vi "Edit a Button--Material.vi"() -> ()   [LabVIEW 2021]
doc: "Edit/create buttons based on a few built-in templates.\n\n<b>Code Developed By:</b>\nTechnology Service Corporation\n1983 S Liberty Drive\nBloomington, IN 47403\nPhone: 812 558-7100\nwww.tsc.com/atcs\n\nDeveloper:\nDaniel Coons"
uses:
  <vilib>/Utility/miscctls.llb/LVPositionTypeDef.ctl
  user32.dll
  Material Theme/Material Theme.lvclass
  Material-Scheme/Material-Scheme.lvclass
panel:
  in  "Color Level":u16(ring) items=["Primary", "Secondary", "Tertiary", "Error", "Primary Fixed", "Secondary Fixed", "Tertiary Fixed"]
  in  "Theme":u16(ring) items=["Light Theme", "Light Medium Contrast", "Light High Contrast", "Dark Theme", "Dark Medium Contrast", "Dark High Constrast"]
  in  "theme path":path
  in  "Open":bool
  in  "Button Type":u16(ring) items=["FAB--icon--rounded.ctl", "filled--icon--rectangular.ctl", "filled--icon--rounded.ctl", "filled--text--rectangular.ctl", "filled--text--rounded.ctl", "nooutline--icon--rectangular--40x40.ctl", "nooutline--icon--rectangular.ctl", "nooutline--icon--rounded.ctl", "nooutline--text--rectangular.ctl", "nooutline--text--rounded.ctl", "outline--icon--rectangular.ctl", "outline--icon--rounded.ctl", "outline--text--rectangular.ctl", "outline--text--rounded.ctl", "tonal--icon--rectangular.ctl", "tonal--icon--rounded.ctl", "tonal--text--rectangular.ctl", "tonal--text--rounded.ctl"]
  in  "Tab Control":enum32{"Button Formatting"}(tab)
  in  "Image Color":u32(colorbox)=3563918
  in  "update button text location":bool
  in  "Button Text Location":cluster{"Left":i32, "Top":i32}
  in  "update button size":bool
  in  "Button Size":cluster{"Width":u32, "Height":u32}={"Width"=204, "Height"=48}
  in  "update colors":bool
  in  "Boolean Text":string
  in  "Boolean Text Format":T1={"Font:Color"=3563918, "Font:Bold?"=TRUE, "Font:Name"="App Font", "Font:Size"=22}
  in  "Boolean Colors":T2={"false color"={"border"=15922170, "fill"=15922170}, "true color"={"border"=14936305, "fill"=14936305}, "click false color"={"border"=14410221, "fill"=14410221}, "click true color"={"border"=14410221, "fill"=14410221}, "hover false color"={"border"=14540516, "fill"=14540516}, "hover true color"={"border"=14540516, "fill"=14540516}}
  in  "update text format":bool
  in  "Decal Image":path
  out "b":u8
  out "g":u8
  out "r":u8
  out "Color":u32(colorbox)
  in  "Hex Color":u32 max=16777215 format="%06x"
  in  "close":bool
  out "header":bool
  in  "Save":bool
  out "error out":errorcluster
  # "if using hex colors, put in the value and copy/paste\nto whichever desired color box"
  # "Note: match the size of the replacement\nimage so scaling is correct (default 24x24)\n\nFor other desired sizes, save the control and\nopen it in LabVIEW. Click the Wrench in the\ntool bar to change to Edit Mode. \n\nRight click the image on the button and \nchoose Original Size.\n\nGetting the right size glyph can be a\nchallenge with customized buttons"
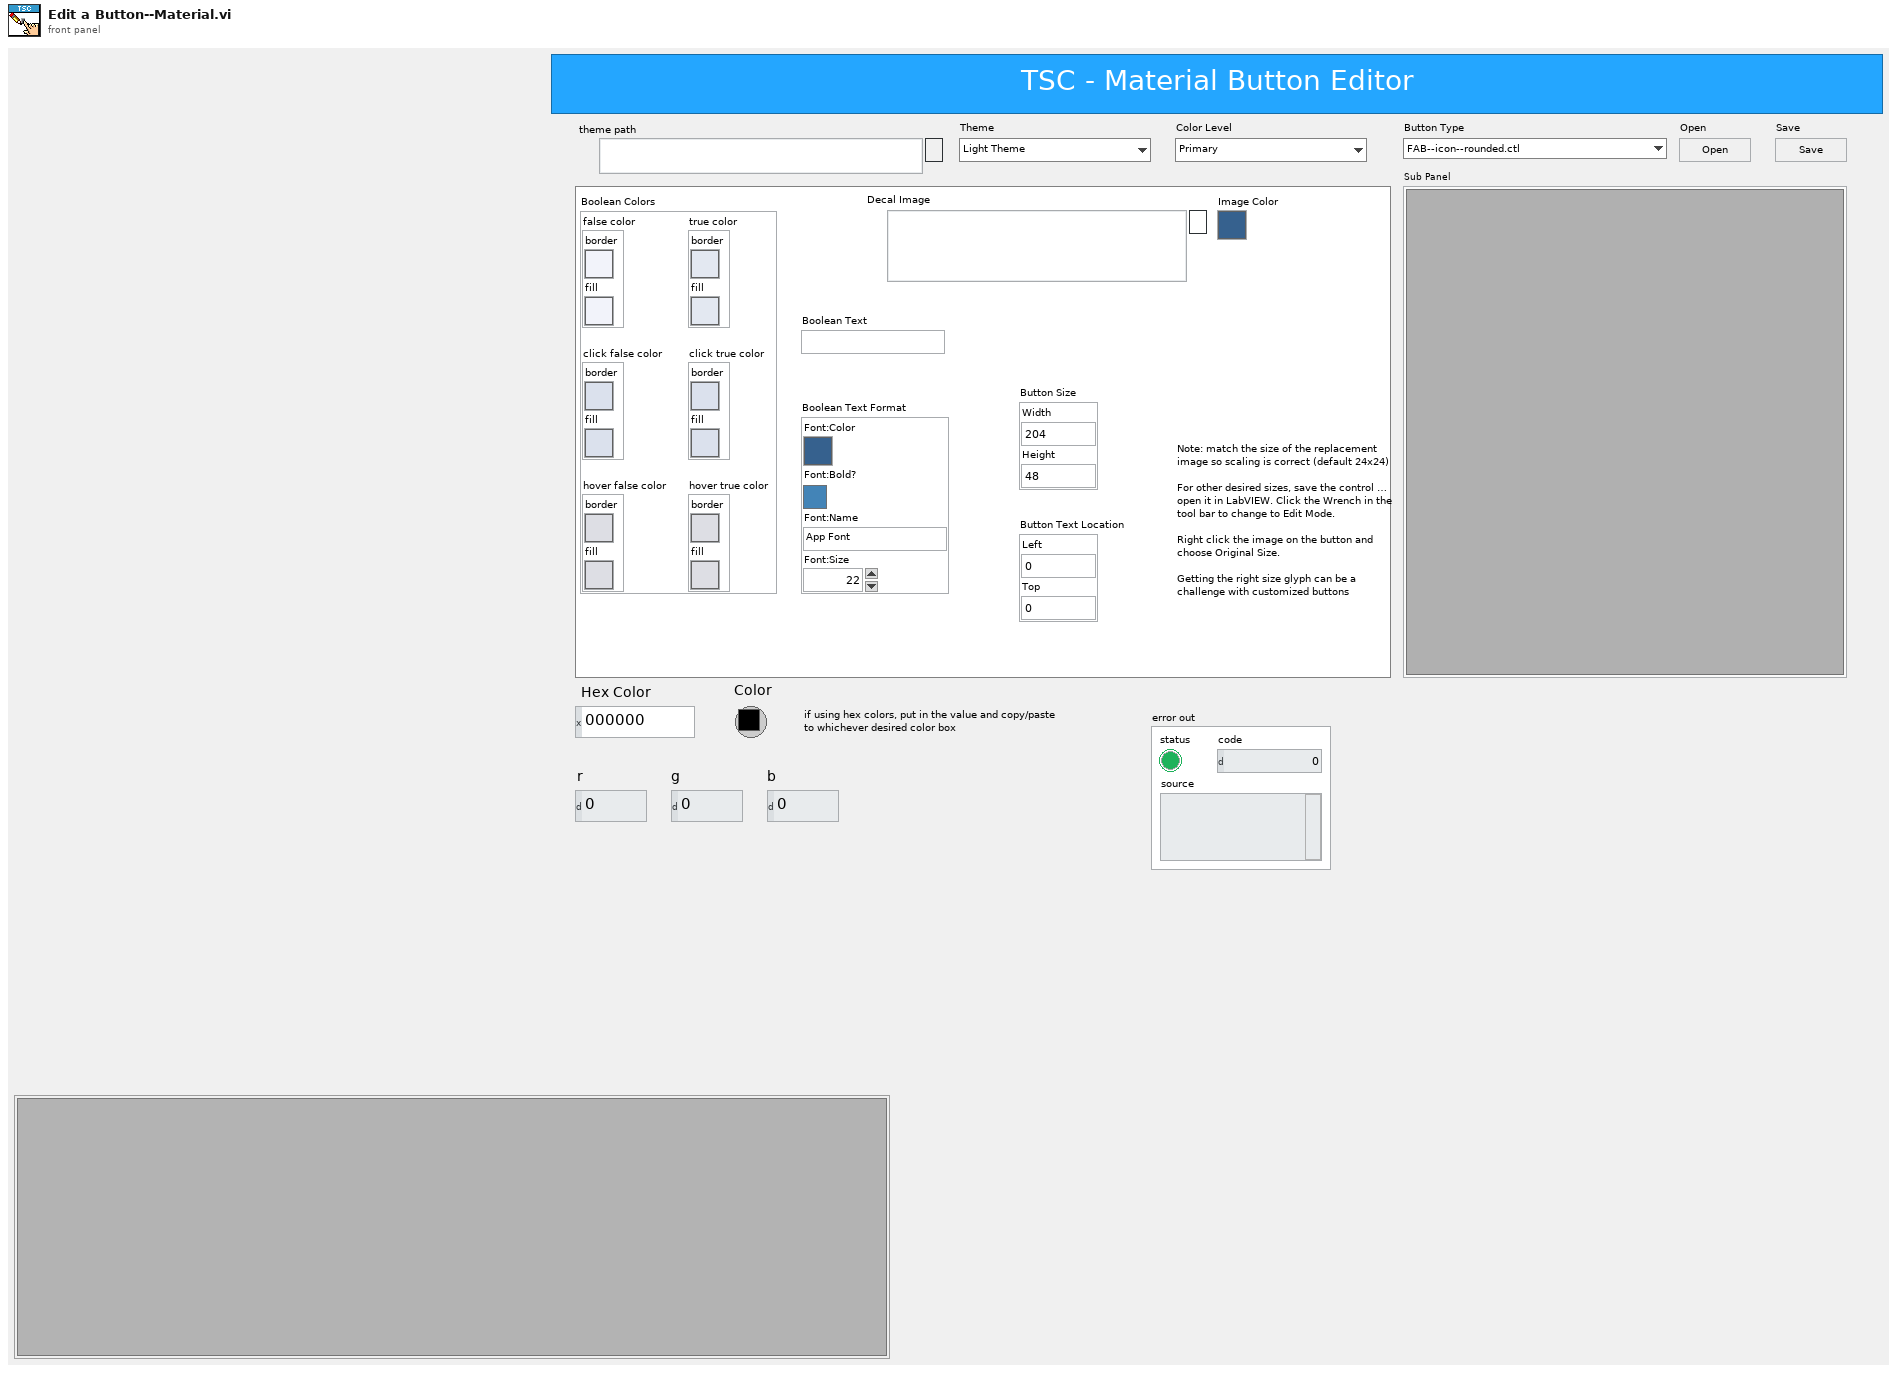
[diagram p1: front panel]
types:
  T1 = cluster{"Font:Color":u32, "Font:Bold?":bool, "Font:Name":string, "Font:Size":u32}
  T2 = cluster{"false color":cluster{"border":u32, "fill":u32}, "true color":cluster{"border":u32, "fill":u32}, "click false color":cluster{"border":u32, "fill":u32}, "click true color":cluster{"border":u32, "fill":u32}, "hover false color":cluster{"border":u32, "fill":u32}, "hover true color":cluster{"border":u32, "fill":u32}}
  T3 = typedef "User Events.ctl" = cluster{"update colors":refnum<user-event>, "update boolean data":refnum<user-event>, "update image":refnum<user-event>}
  T4 = typedef "LVPositionTypeDef.ctl" = cluster{"Left":i32, "Top":i32}
  T5 = enum32{"invalid VI type", "Standard VI", "Control VI", "Global VI", "Polymorphic VI", "Configuration VI", "SubSystem", "Facade VI", "Method VI", "Statechart Diagram VI"}
  T6 = typedef "LVBoundsTypeDef.ctl" = cluster{"Width":u32, "Height":u32}
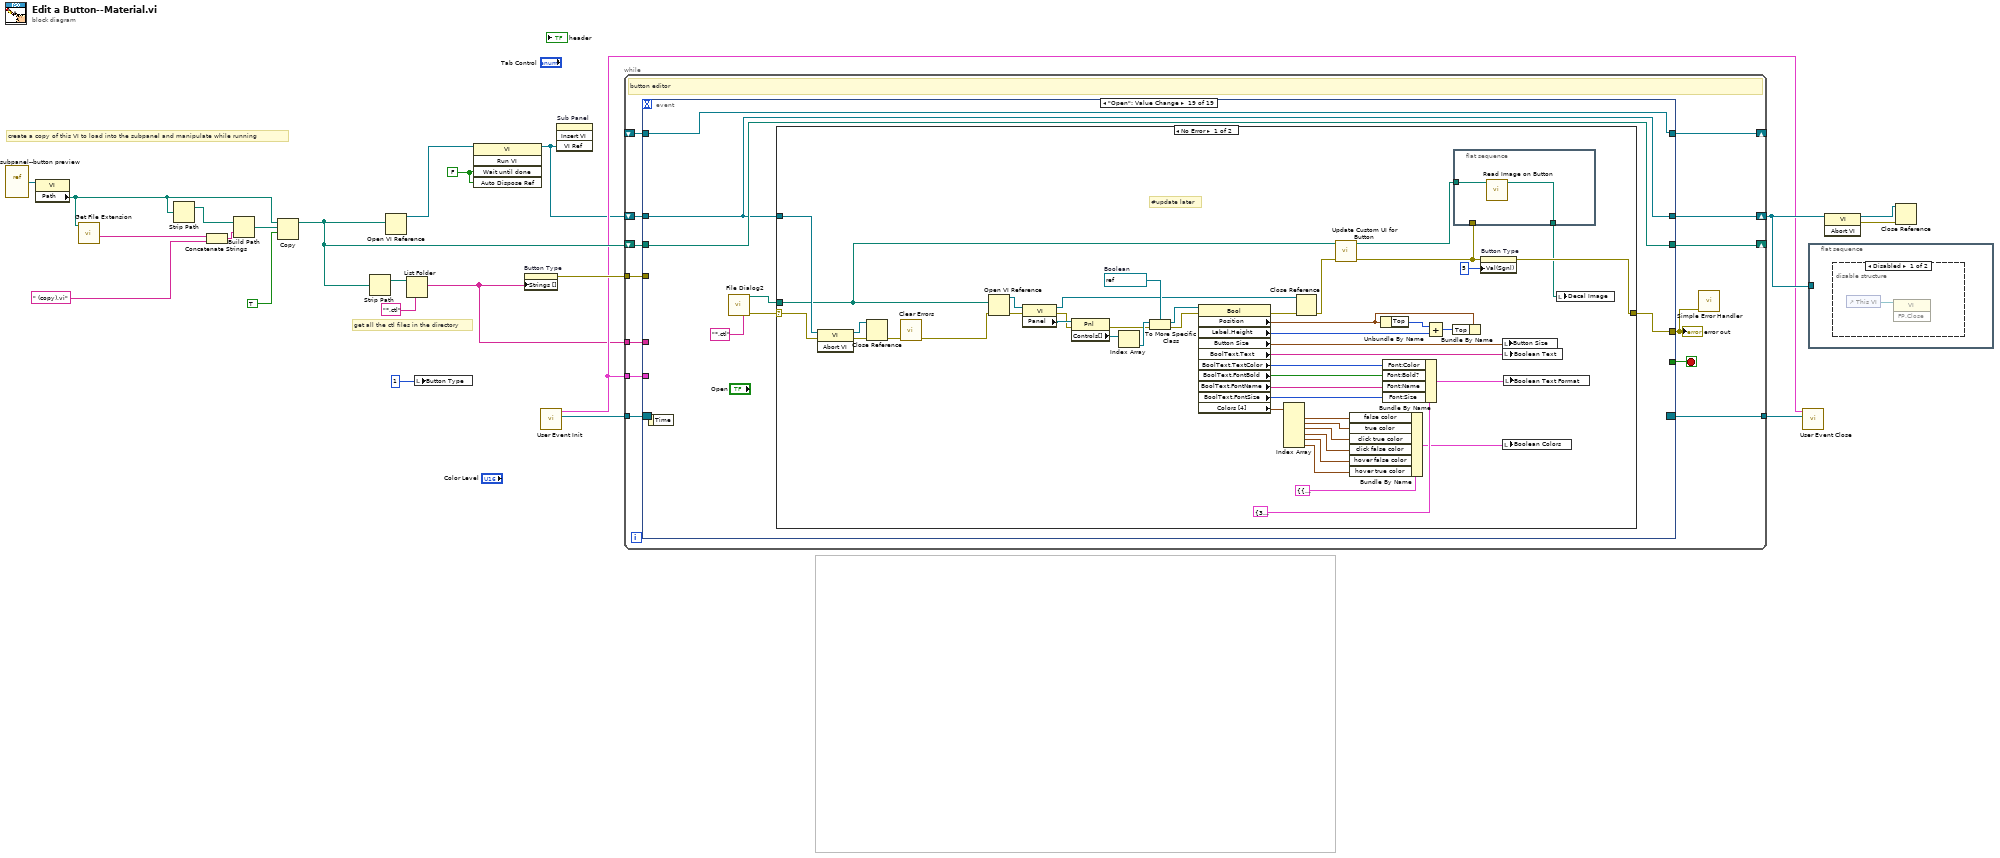
[diagram p0: block diagram]
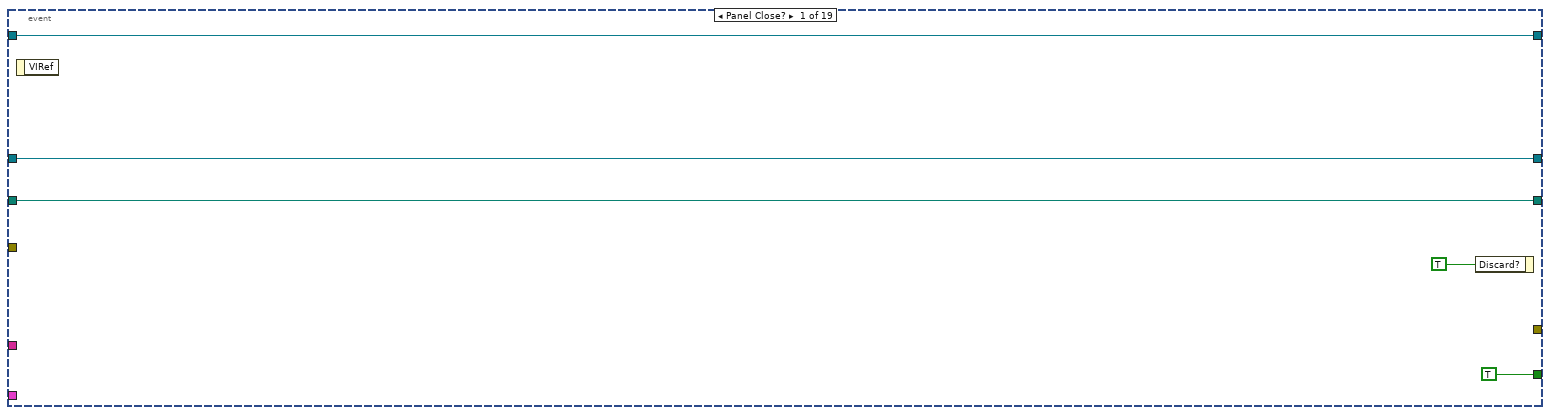
[diagram p3: hidden frame]
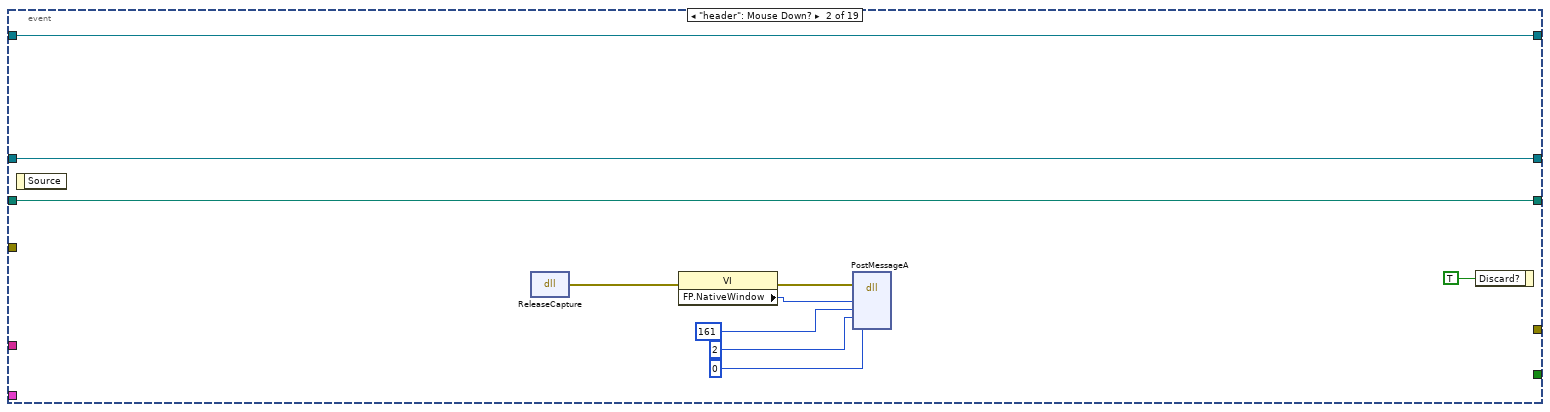
[diagram p4: hidden frame]
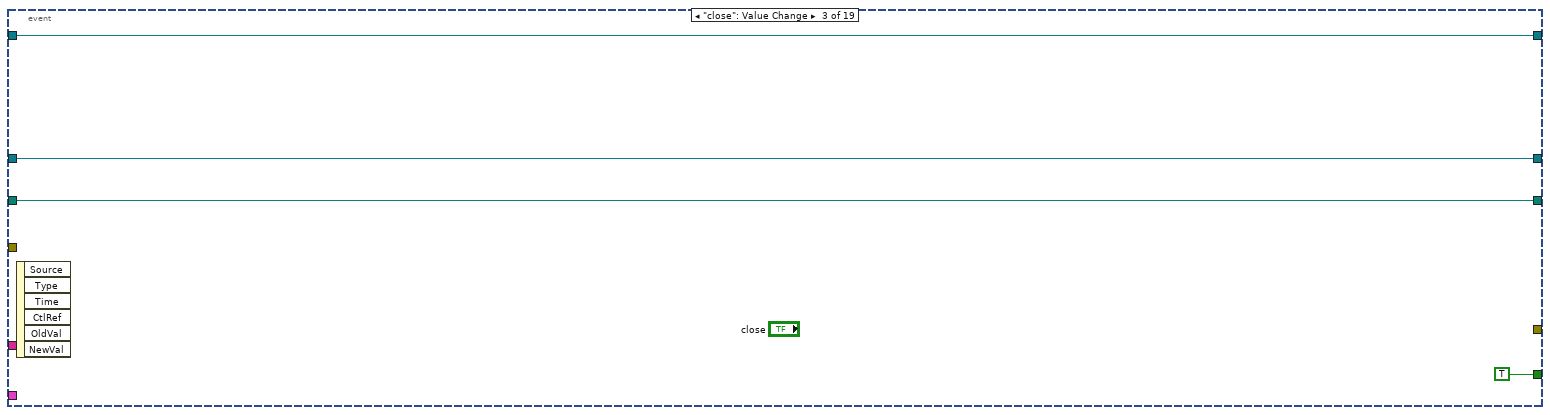
[diagram p5: hidden frame]
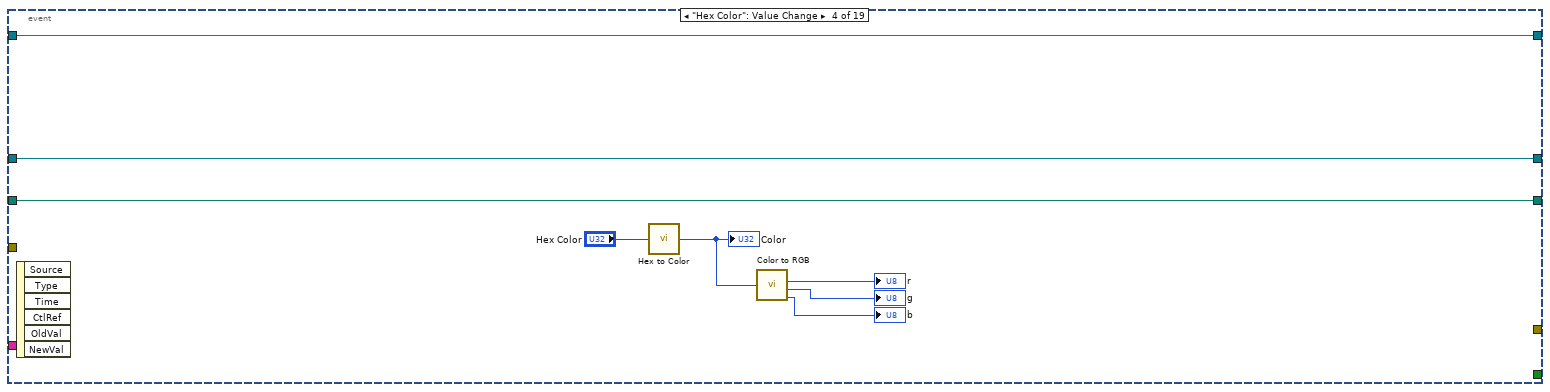
[diagram p6: hidden frame]
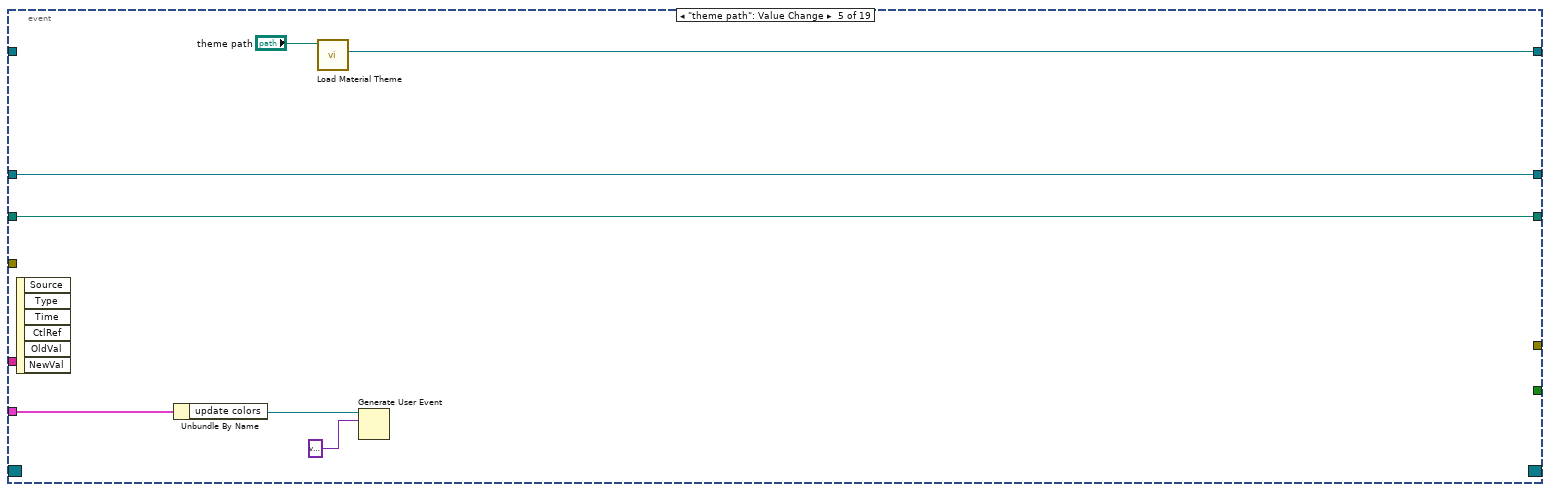
[diagram p7: hidden frame]
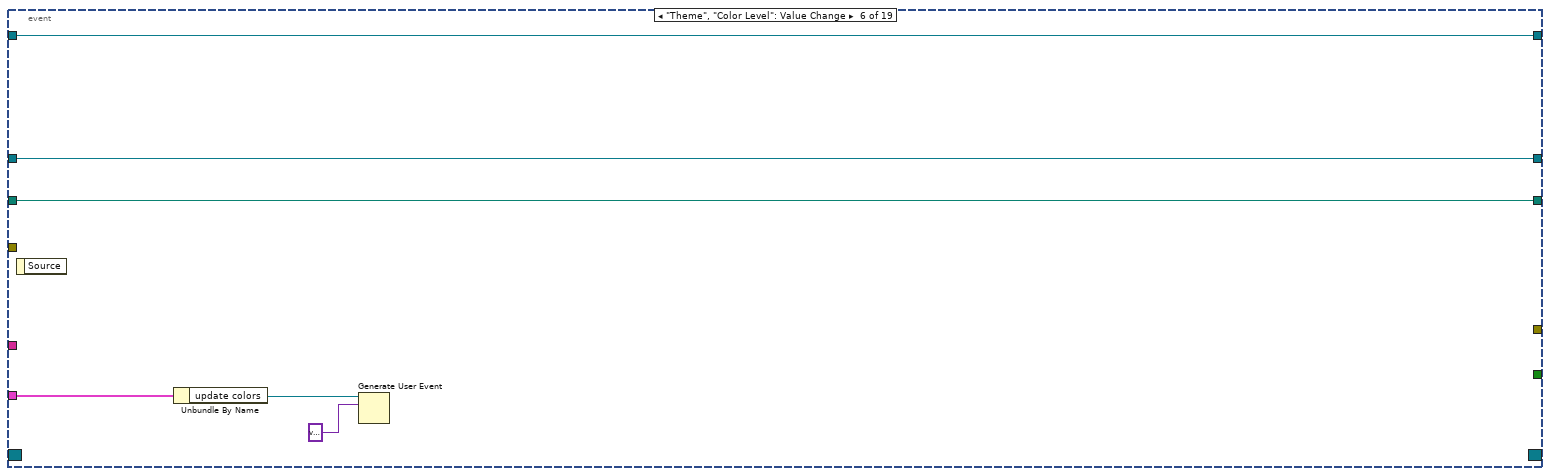
[diagram p8: hidden frame]
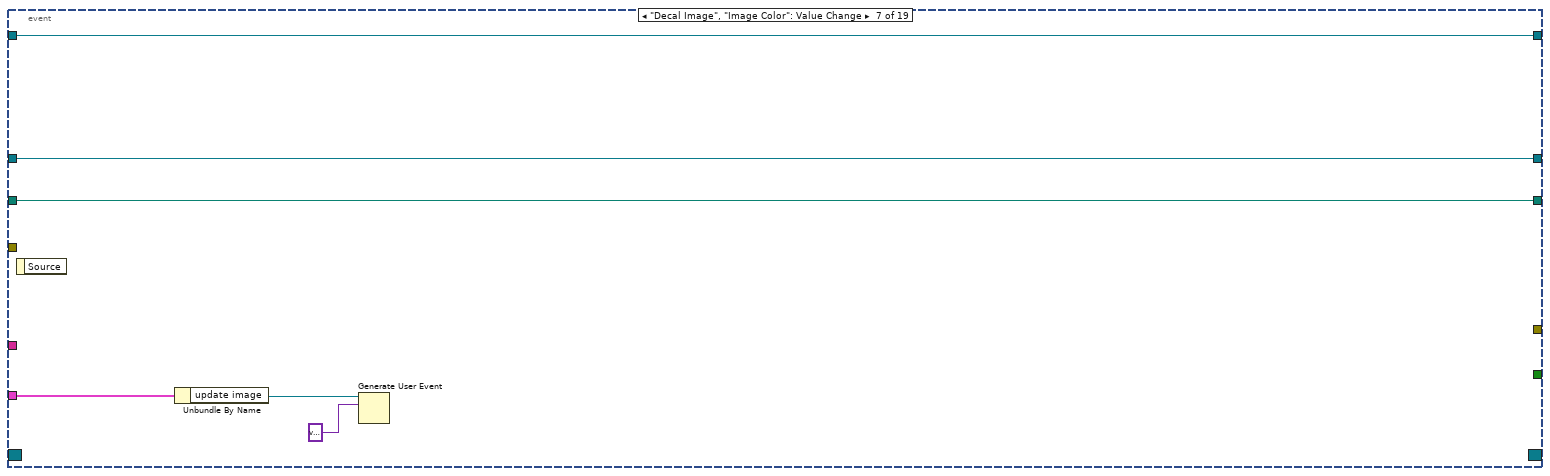
[diagram p9: hidden frame]
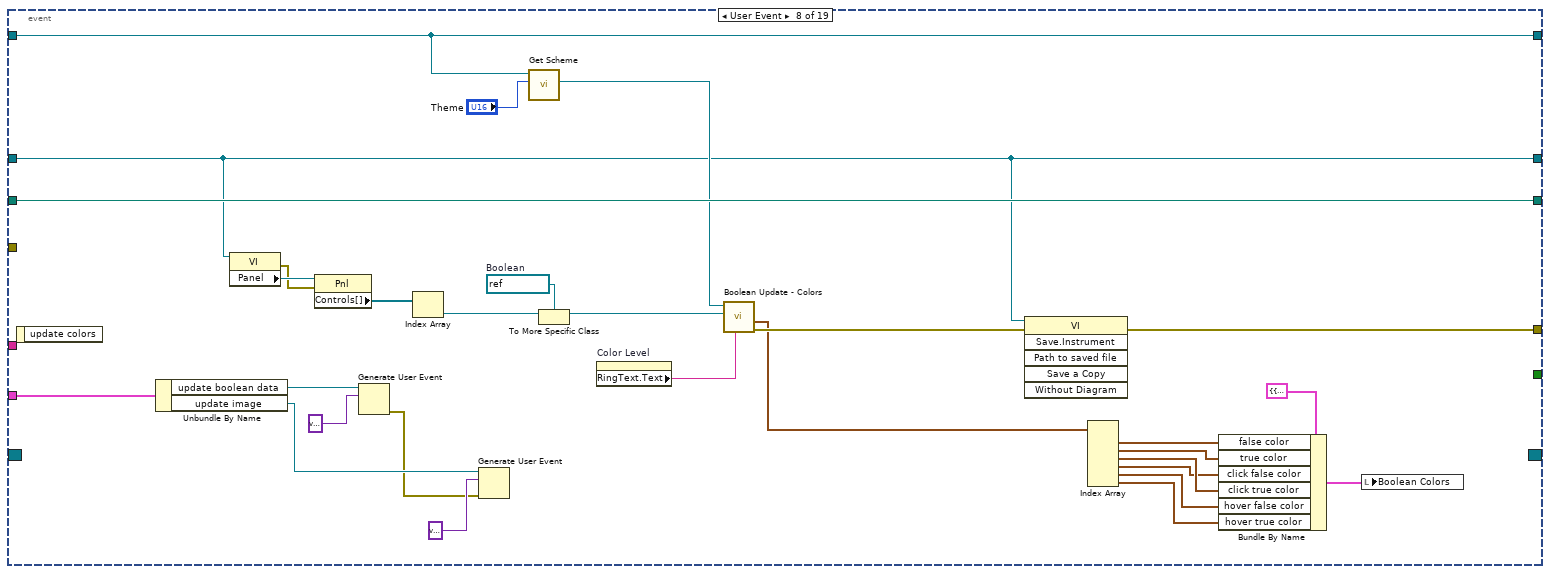
[diagram p10: hidden frame]
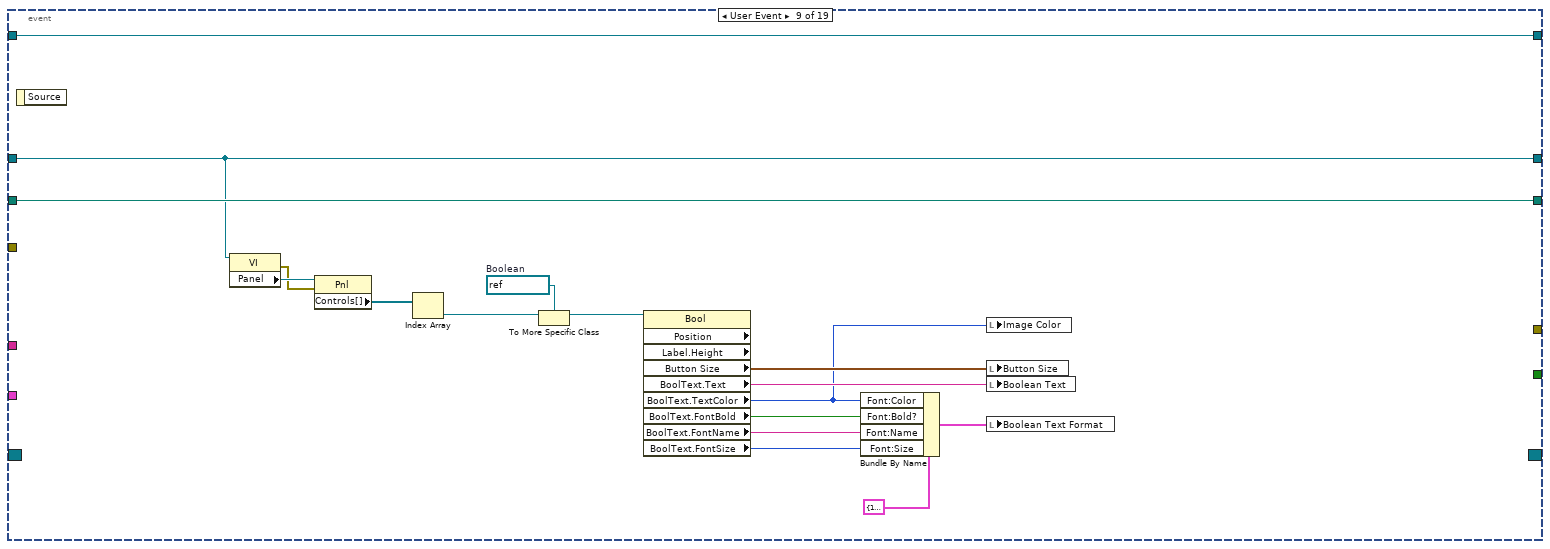
[diagram p11: hidden frame]
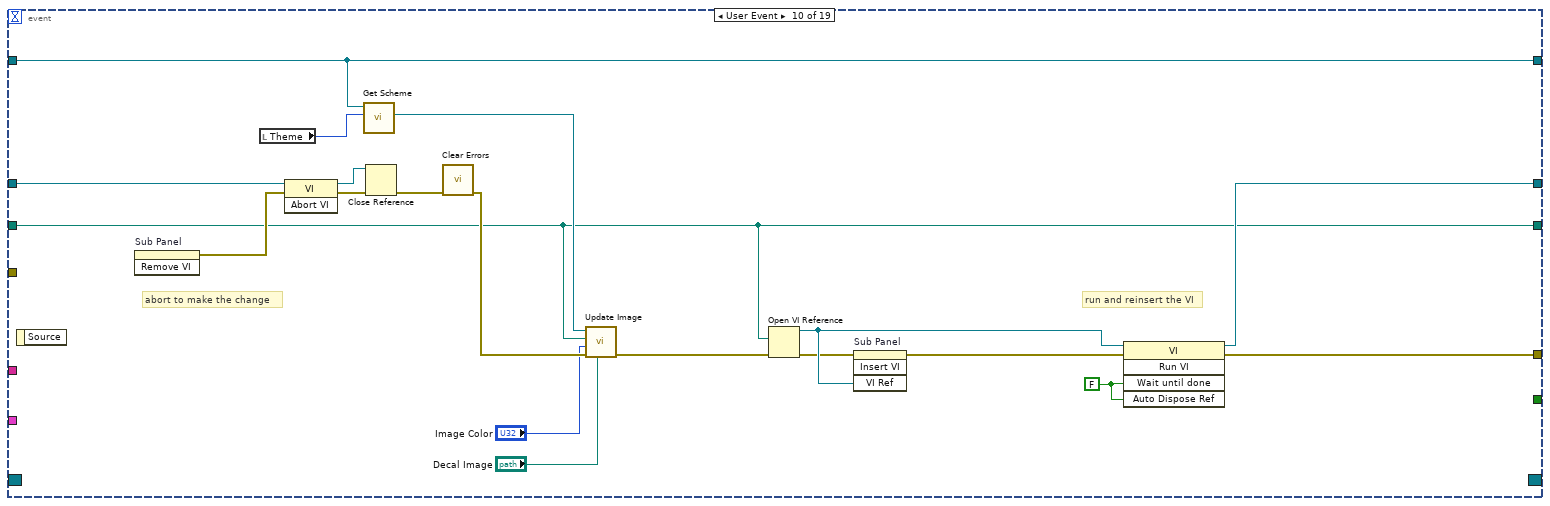
[diagram p12: hidden frame]
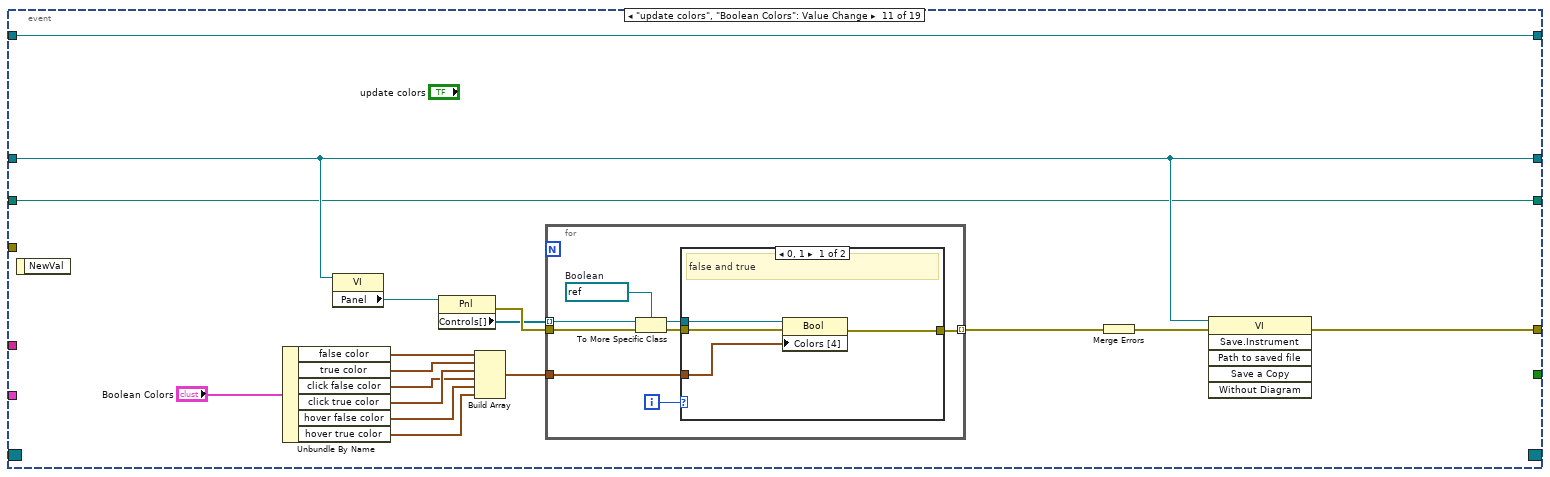
[diagram p13: hidden frame]
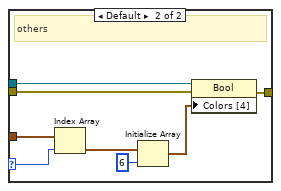
[diagram p14: hidden frame]
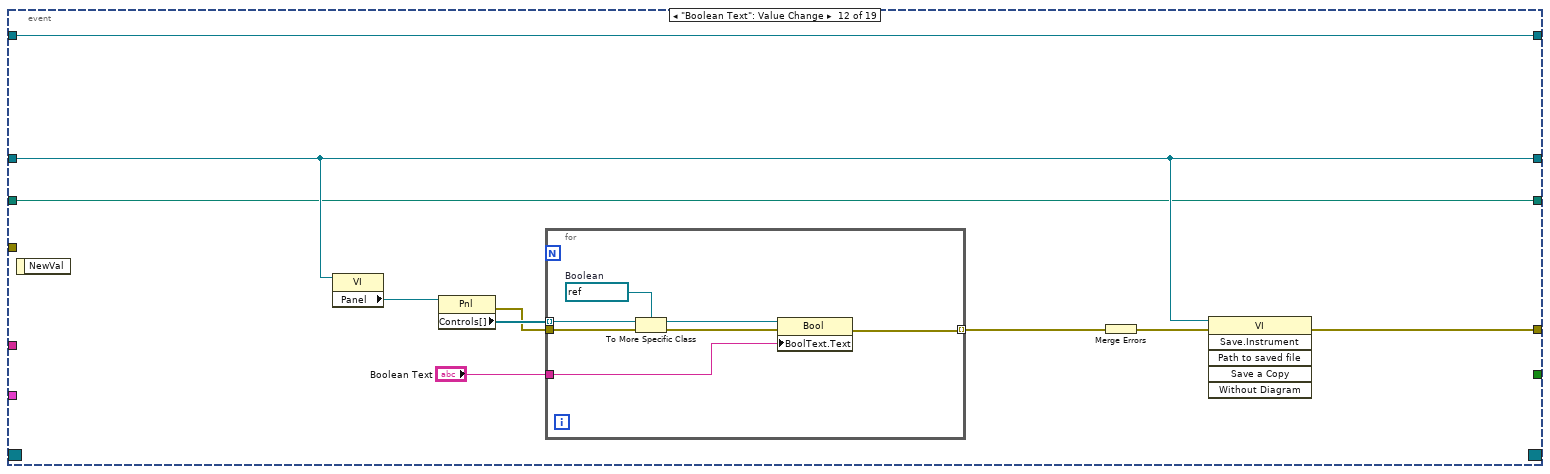
[diagram p15: hidden frame]
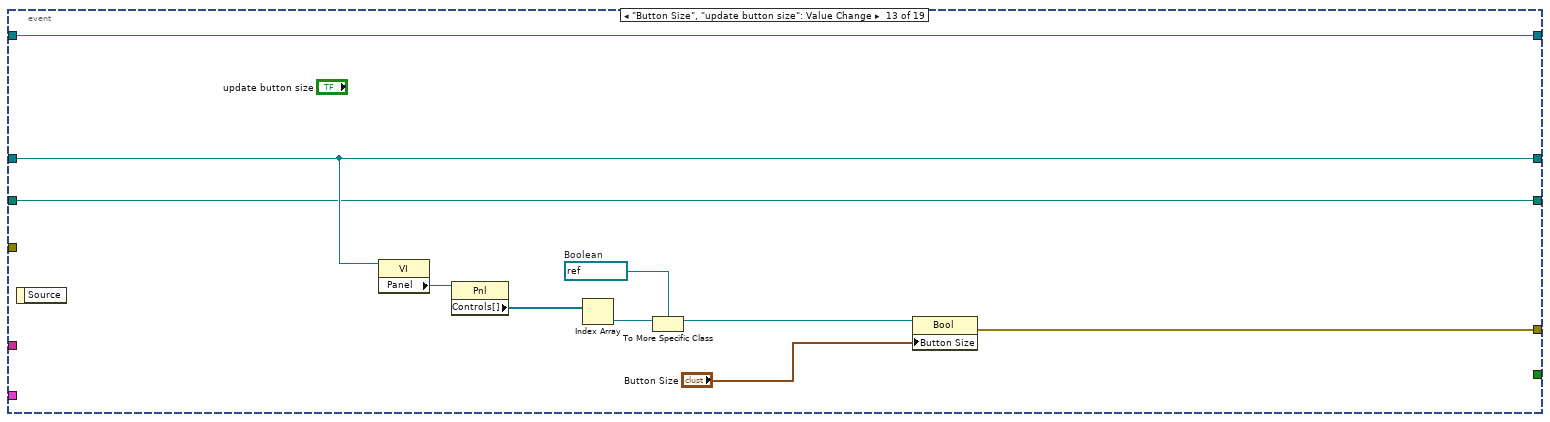
[diagram p16: hidden frame]
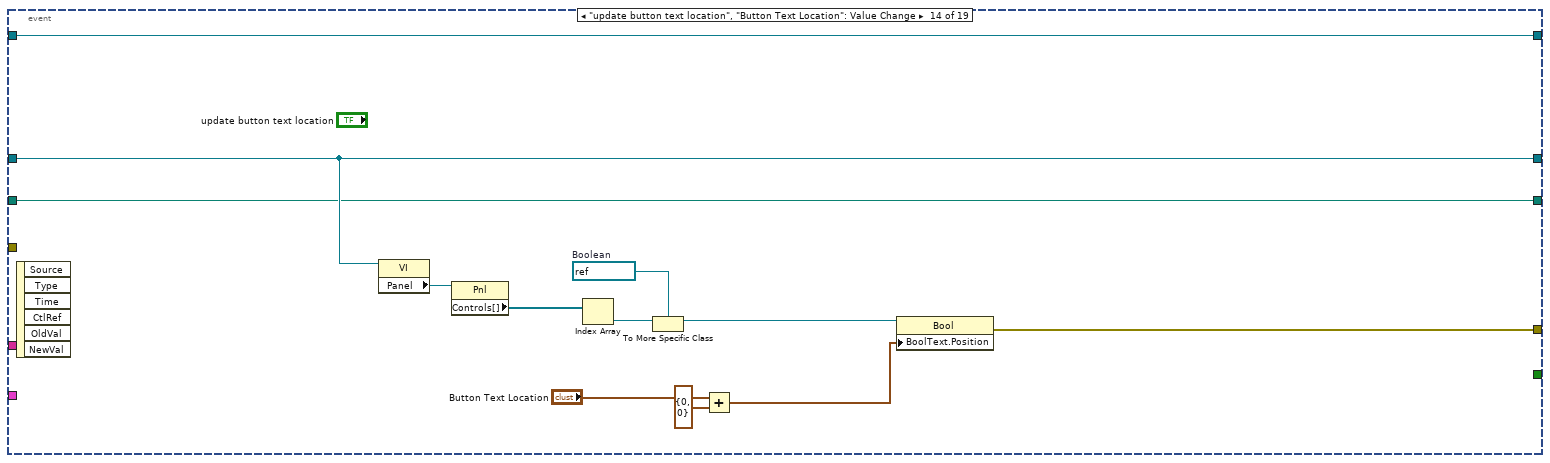
[diagram p17: hidden frame]
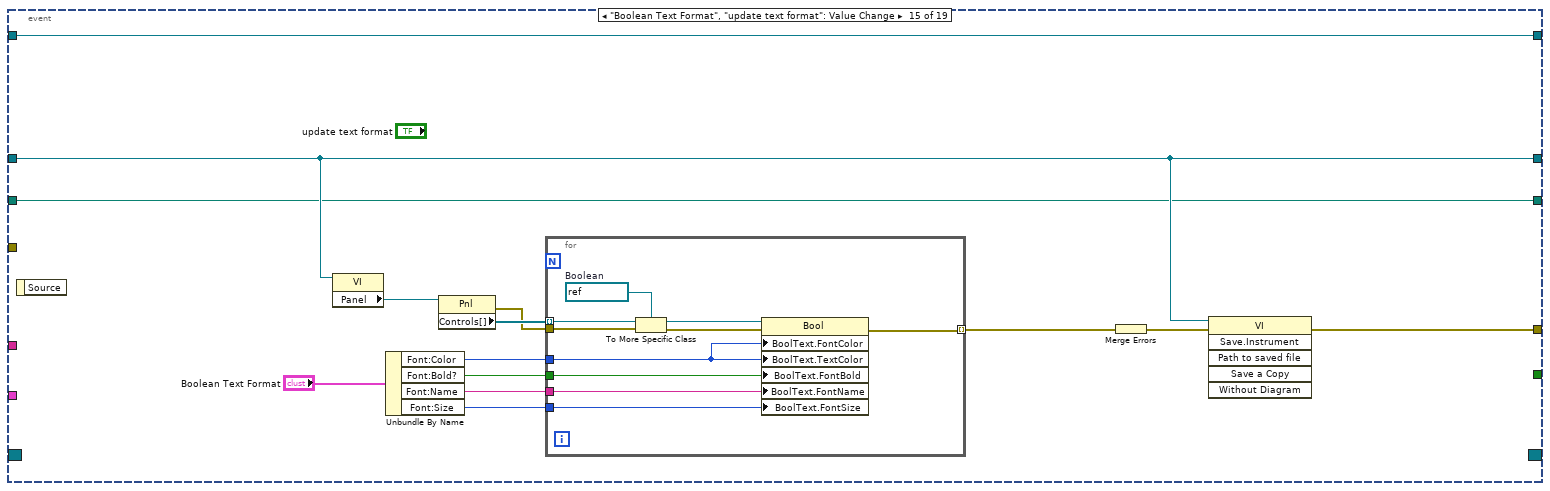
[diagram p18: hidden frame]
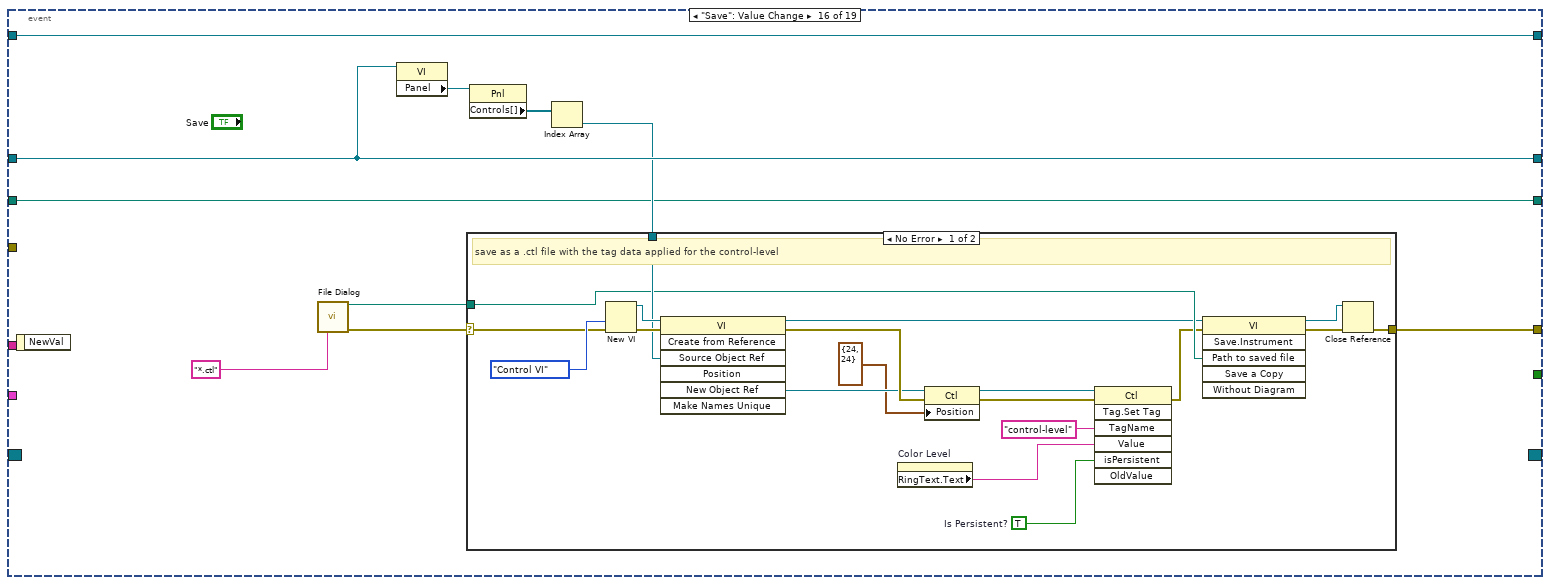
[diagram p19: hidden frame]
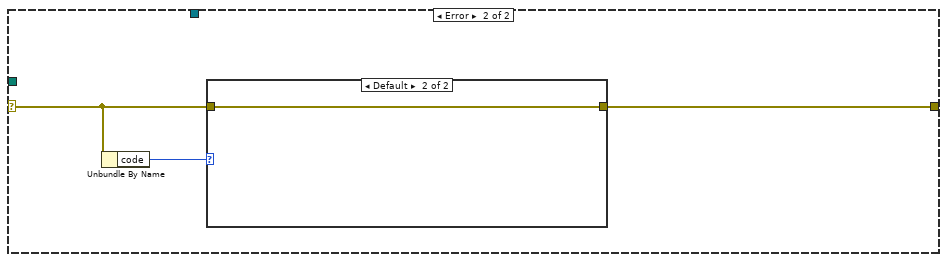
[diagram p20: hidden frame]
diagram:
  w12 = FALSE ("Activate?")
  # "get all the ctl files in the directory"
  # "create a copy of this VI to load into the subpanel and manipulate while running"
  n1 = vi-ref "subpanel--button preview.vi"() -> (w10:refnum<vi>)
  n2 = property class="VI"(reference=w10) -> ("Path"=w3:path)  [unwired: 1 in, 2 out]
  n3 = call <vilib>:"Get File Extension.vi"("file"=w3) -> ("filename without extension"=w4:string)  [unwired: 6 in, 4 out]
  n4 = Strip Path(path=w3) -> (stripped path=w6:path)  [unwired: 1 out]
  n5 = Concatenate Strings(w4, " (copy).vi" ("string")) -> (w7:string)
  n6 = Build Path(base path=w6, name or relative path=w7) -> (appended path=w5:path)
  n7 = Copy(9:TRUE ("overwrite (F)"), 10:w5, 11:w3) -> (3:w17:path)  [unwired: 2 in, 2 out]
  n8 = Strip Path(path=w17) -> (stripped path=w18:path)  [unwired: 1 out]
  n9 = Open VI Reference(vi path=w17) -> (vi reference=w16:refnum<vi>)  [unwired: 5 in, 1 out]
  n10 = List Folder(path=w18, pattern="*.ctl") -> (filenames=w11:string[])  [unwired: 2 in, 3 out]
  n11 = local write "Button Type"(1) -> ()
  n12 = invoke class="VI" method="Run VI"(reference=w16, "Wait until done"=w12, "Auto Dispose Ref"=w12) -> (reference out=w1:refnum<vi>)  [unwired: 2 in, 4 out]
  n13 = property on="Button Type" class="Ring (strict)"("Strings []"=w11) -> (error out=w21:errorcluster)  [unwired: 2 in, 1 out]
  n14 = call "User Event Init.vi"() -> ("Event Registration Refnum"=w15:refnum<event-registration>, "user events"=w13:T3)  [unwired: 10 in]
  n15 = invoke on="Sub Panel" class="SubPnl" method="Insert VI"("VI Ref"=w1) -> ()  [unwired: 3 in, 4 out]
  n16 = while {
    shift-right: [w34] -> w20
    shift-left: w1 -> [w35]
    shift-right: [w32] -> _
    shift-left: w17 -> [w33]
    tunnel: w21 -> [w31]
    shift-right: [w30] -> _
    shift-left: _ -> [w29]
    tunnel: w15 -> [w28]
    tunnel: [w27] -> w14
    tunnel: w13 -> [w26]
    tunnel: w11 -> [w25]
    stop <- w36 stop-if-true
    # "button editor"
    n17 = event shown="[18] \"Open\": Value Change" {
      selector: w28 -> [_ _ _ _ _ _ _ _ _ _ _ _ _ _ _ _ _ _ _]
      dyn-events: [_ _ _ _ _ _ _ _ _ _ _ _ _ _ _ _ _ _ _] -> w27
      timeout: _ -> [_ _ _ _ _ _ _ _ _ _ _ _ _ _ _ _ _ _ _]
      tunnel: [TRUE _ TRUE _ _ _ _ _ _ _ _ _ _ _ _ _ _ _ _] -> w36
      tunnel: w35 -> [w39 w51 w54 w63 w67 w75 w81 w88 w121 w147 w160 w187 w207 w219 w231 w256 w285 w339 w350]
      tunnel: [w39 w51 w54 w63 w67 w75 w81 w88 w121 w140 w160 w187 w207 w219 w231 w256 w285 w332 w350] -> w34
      tunnel: [_ _ _ _ _ _ _ w86 _ w129 w159 w188 w205 w217 w232 w253 w284 w333 w352] -> w24
      tunnel: w33 -> [w38 w43 w53 w57 w70 w76 w82 w111 w128 w131 w149 w186 w203 w214 w225 w249 w283 w331 w355]
      tunnel: [w38 w43 w53 w57 w70 w76 w82 w111 w128 w131 w149 w186 w203 w214 w225 w249 w283 w331 w355] -> w32
      tunnel: w31 -> [_ _ _ _ _ _ _ _ _ _ _ _ _ _ _ _ _ _ _]
      tunnel: [w37 w42 w52 w56 w68 w72 w78 w102 w127 w144 w148 w185 w202 w213 w224 w248 w282 w337 w349] -> w30
      tunnel: w29 -> [w37 w42 w52 w56 _ w72 w78 w102 w127 w144 w148 w185 w202 w213 w224 w248 w282 w337 w349]
      tunnel: w26 -> [_ _ _ _ w66 w74 w80 w89 _ _ _ _ _ _ _ _ _ w319 _]
      tunnel: w25 -> [_ _ _ _ _ _ _ _ _ _ _ _ _ _ _ _ _ _ _]
      event Panel Close? {
        n18 = event-data() -> ()  [unwired: 1 in, 1 out]
        n19 = event-data("Discard?"=TRUE) -> ()  [unwired: 1 in, 1 out]
      }
      event "header": Mouse Down? {
        n20 = event-data() -> ()  [unwired: 1 in, 1 out]
        n21 = dll-call lib="user32.dll" fn="ReleaseCapture"() -> (error out=w46:errorcluster)  [unwired: 4 in, 1 out]
        n22 = property class="VI"(error in=w46) -> (error out=w45:errorcluster, "FP.NativeWindow"=w44:u64)  [unwired: 1 in, 1 out]
        n23 = dll-call lib="user32.dll" fn="PostMessageA"(error in=w45, "hWnd"=w44, "Msg"=161, "wParam"=2, "lParam"=0) -> ()  [unwired: 7 in, 2 out]
        n24 = event-data("Discard?"=TRUE) -> ()  [unwired: 1 in, 1 out]
      }
      event "close": Value Change {
        n25 = event-data() -> ()  [unwired: 1 in, 6 out]
      }
      event "Hex Color": Value Change {
        n26 = event-data() -> ()  [unwired: 1 in, 6 out]
        n27 = call <vilib>:"Hex to Color.vi"("Hex String"="Hex Color") -> ("Color Box"=w61:u32)  [unwired: 4 in]
        "Color" <- w61
        n28 = call <vilib>:"Color to RGB.vi"("Color"=w61) -> ("R"=→"r":u8, "G"=→"g":u8, "B"=→"b":u8)  [unwired: 1 out]
      }
      event "theme path": Value Change {
        n29 = event-data() -> ()  [unwired: 1 in, 6 out]
        n30 = Unbundle By Name(w66) -> ("update colors"=w64:refnum<user-event>)
        n31 = call "Load Material Theme.vi"("file path (use dialog)"="theme path") -> ("Theme"=w68:refnum<class "Material Theme.lvclass">)  [unwired: 9 in, 1 out]
        n32 = Generate User Event(user event=w64, event data cluster=variant ("event data")) -> ()  [unwired: 2 in, 2 out]
      }
      event "Theme", "Color Level": Value Change {
        n33 = event-data() -> ()  [unwired: 1 in, 1 out]
        n34 = Unbundle By Name(w74) -> ("update colors"=w71:refnum<user-event>)
        n35 = Generate User Event(user event=w71, event data cluster=variant ("event data")) -> ()  [unwired: 2 in, 2 out]
      }
      event "Decal Image", "Image Color": Value Change {
        n36 = event-data() -> ()  [unwired: 1 in, 1 out]
        n37 = Unbundle By Name(w80) -> ("update image"=w77:refnum<user-event>)
        n38 = Generate User Event(user event=w77, event data cluster=variant ("event data")) -> ()  [unwired: 2 in, 2 out]
      }
      event User Event {
        w105 = refnum<vi> refnum  # Boolean
        n39 = event-data() -> ()  [unwired: 1 in, 1 out]
        n40 = Unbundle By Name(w89) -> ("update boolean data"=w91:refnum<user-event>, "update image"=w84:refnum<user-event>)
        n41 = property class="VI"(reference=w88) -> (error out=w107:errorcluster, "Panel"=w110:refnum<vi>)  [unwired: 1 in, 1 out]
        n42 = property class="Pnl"(reference=w110, error in=w107) -> ("Controls[]"=w109:refnum<vi>[])  [unwired: 2 out]
        n43 = Generate User Event(user event=w91, event data cluster=variant ("event data")) -> (error out=w83:errorcluster)  [unwired: 2 in, 1 out]
        n44 = Index Array(array=w109) -> (element=w108:refnum<vi>)  [unwired: 1 in]
        n45 = Generate User Event(user event=w84, event data cluster=variant ("event data"), error in=w83) -> ()  [unwired: 1 in, 2 out]
        n46 = call "Get Scheme.vi"("Theme"="Theme", "Material Theme in"=w102) -> ("Material-Scheme"=w104:refnum<class "Material-Scheme.lvclass">)  [unwired: 7 in, 2 out]
        n47 = To More Specific Class(target class=w105, reference=w108) -> (specific class reference=w106:refnum<vi>)  [unwired: 1 in, 1 out]
        n48 = property on="Color Level" class="Ring (strict)"() -> ("RingText.Text"=w87:string)  [unwired: 2 in, 2 out]
        n49 = call "Boolean Update - Colors.vi"("control-level"=w87, "Bool Refnum"=w106, "Material-Scheme in"=w104) -> ("error out"=w103:errorcluster, "Array"=w100:cluster{"bg":u32, "fg":u32}[])  [unwired: 5 in, 2 out]
        n50 = invoke class="VI" method="Save.Instrument"(reference=w88, error in=w103) -> (error out=w86:errorcluster)  [unwired: 4 in, 5 out]
        n51 = Index Array(array=w100) -> (element #1=w98:cluster{"bg":u32, "fg":u32}, element #2=w97:cluster{"bg":u32, "fg":u32}, element #3=w96:cluster{"bg":u32, "fg":u32}, element #4=w95:cluster{"bg":u32, "fg":u32}, element #5=w94:cluster{"bg":u32, "fg":u32}, element #6=w93:cluster{"bg":u32, "fg":u32})  [unwired: 6 in]
        n52 = Bundle By Name(cluster=T2 {"false color"={"border"=15922170, "fill"=15922170}, "true color"={"border"=14936305, "fill"=14936305}, "click false color"={"border"=14410221, "fill"=14410221}, "click true color"={"border"=14410221, "fill"=14410221}, "hover false color"={"border"=14540516, "fill"=14540516}, "hover true color"={"border"=14540516, "fill"=14540516}} ("Boolean Colors"), "false color"=w98, "true color"=w97, "click false color"=w95, "click true color"=w96, "hover false color"=w94, "hover true color"=w93) -> (w92:T2)
        n53 = local write "Boolean Colors"(w92) -> ()
      }
      event User Event {
        w122 = refnum<vi> refnum  # Boolean
        n54 = event-data() -> ()  [unwired: 1 in, 1 out]
        n55 = property class="VI"(reference=w121) -> (error out=w123:errorcluster, "Panel"=w126:refnum<vi>)  [unwired: 1 in, 1 out]
        n56 = property class="Pnl"(reference=w126, error in=w123) -> ("Controls[]"=w125:refnum<vi>[])  [unwired: 2 out]
        n57 = Index Array(array=w125) -> (element=w124:refnum<vi>)  [unwired: 1 in]
        n58 = To More Specific Class(target class=w122, reference=w124) -> (specific class reference=w120:refnum<vi>)  [unwired: 1 in, 1 out]
        n59 = property class="Bool" props=["Position", "Label", "Height", "Button Size", "BoolText", "Text", "BoolText", "TextColor", "BoolText", "FontBold", "BoolText", "FontName", "BoolText", "FontSize"](reference=w120) -> ("Button Size"=w119:T6, "BoolText.Text"=w117:string, "BoolText.TextColor"=w112:u32, "BoolText.FontBold"=w116:bool, "BoolText.FontName"=w115:string, "BoolText.FontSize"=w114:u32)  [unwired: 1 in, 4 out]
        n60 = Bundle By Name(cluster=T1 {"Font:Color"=13140, "Font:Bold?"=TRUE, "Font:Name"="App Font", "Font:Size"=22} ("Boolean Text Format"), "Font:Color"=w112, "Font:Bold?"=w116, "Font:Name"=w115, "Font:Size"=w114) -> (w113:T1)
        n61 = local write "Image Color"(w112) -> ()
        n62 = local write "Button Size"(w119) -> ()
        n63 = local write "Boolean Text"(w117) -> ()
        n64 = local write "Boolean Text Format"(w113) -> ()
      }
      event User Event {
        w145 = FALSE ("Wait Until Done")
        # "run and reinsert the VI"
        # "abort to make the change"
        n65 = event-data() -> ()  [unwired: 1 in, 1 out]
        n66 = invoke on="Sub Panel" class="SubPnl" method="Remove VI"() -> (error out=w136:errorcluster)  [unwired: 3 in, 2 out]
        n67 = local read "Theme"() -> (w143:u16)
        n68 = invoke class="VI" method="Abort VI"(reference=w147, error in=w136) -> (reference out=w141:refnum<vi>, error out=w146:errorcluster)  [unwired: 1 in, 1 out]
        n69 = call "Get Scheme.vi"("Theme"=w143, "Material Theme in"=w144) -> ("Material-Scheme"=w137:refnum<class "Material-Scheme.lvclass">)  [unwired: 7 in, 2 out]
        n70 = Close Reference(reference=w141, error in (no error)=w146) -> (error out=w142:errorcluster)
        n71 = call <vilib>:"Clear Errors.vi"("error in (no error)"=w142) -> ("error out"=w139:errorcluster)  [unwired: 5 in, 1 out]
        n72 = call "Update Image.vi"("Replace Image"="Decal Image", "error in"=w139, "New Color"="Image Color", "New Control"=w131, "Material-Scheme.lvclass"=w137) -> ("error out"=w138:errorcluster)  [unwired: 5 in, 1 out]
        n73 = Open VI Reference(vi path=w131, error in (no error)=w138) -> (vi reference=w134:refnum<vi>, error out=w133:errorcluster)  [unwired: 4 in]
        n74 = invoke on="Sub Panel" class="SubPnl" method="Insert VI"(error in=w133, "VI Ref"=w134) -> (error out=w132:errorcluster)  [unwired: 2 in, 3 out]
        n75 = invoke class="VI" method="Run VI"(reference=w134, error in=w132, "Wait until done"=w145, "Auto Dispose Ref"=w145) -> (reference out=w140:refnum<vi>, error out=w129:errorcluster)  [unwired: 1 in, 3 out]
      }
      event "update colors", "Boolean Colors": Value Change {
        n76 = event-data() -> ()  [unwired: 1 in, 1 out]
        n77 = Unbundle By Name("Boolean Colors") -> ("false color"=w157:cluster{"border":u32, "fill":u32}, "true color"=w156:cluster{"border":u32, "fill":u32}, "click false color"=w154:cluster{"border":u32, "fill":u32}, "click true color"=w155:cluster{"border":u32, "fill":u32}, "hover false color"=w153:cluster{"border":u32, "fill":u32}, "hover true color"=w152:cluster{"border":u32, "fill":u32})
        n78 = property class="VI"(reference=w160) -> ("Panel"=w164:refnum<vi>)  [unwired: 1 in, 2 out]
        n79 = property class="Pnl"(reference=w164) -> (error out=w162:errorcluster, "Controls[]"=w150:refnum<vi>[])  [unwired: 1 in, 1 out]
        n80 = Build Array(w157, w156, w155, w154, w153, w152) -> (w151:cluster{"border":u32, "fill":u32}[])
        n81 = for {
          tunnel: w150 -> [w172] mode=indexing
          tunnel: w151 -> [w169]
          tunnel: w162 -> [w167]
          tunnel: [w168] -> w163 mode=indexing
          i -> [w165]
          w170 = refnum<vi> refnum  # Boolean
          n82 = To More Specific Class(target class=w170, reference=w172, error in=w167) -> (specific class reference=w171:refnum<vi>, error out=w166:errorcluster)
          n83 = case shown="0, 1" w165 {
            selector: w165 -> [_ w180]
            tunnel: w171 -> [w176 w184]
            tunnel: w169 -> [w175 w181]
            tunnel: [w174 w183] -> w168
            tunnel: w166 -> [w173 w182]
            frame 0, 1 {
              # "false and true"
              n84 = property class="Bool"(reference=w176, error in=w173, "Colors [4]"=w175) -> (error out=w174:errorcluster)  [unwired: 1 out]
            }
            frame Default {
              # "others"
              n85 = Index Array(array=w181, index=w180) -> (element=w179:cluster{"border":u32, "fill":u32})
              n86 = Initialize Array(w179, 6 ("dimension size")) -> (w177:cluster{"border":u32, "fill":u32}[])
              n87 = property class="Bool"(reference=w184, error in=w182, "Colors [4]"=w177) -> (error out=w183:errorcluster)  [unwired: 1 out]
            }
          }
        }
        n88 = Merge Errors(w163) -> (w161:errorcluster)
        n89 = invoke class="VI" method="Save.Instrument"(reference=w160, error in=w161) -> (error out=w159:errorcluster)  [unwired: 4 in, 5 out]
      }
      event "Boolean Text": Value Change {
        n90 = event-data() -> ()  [unwired: 1 in, 1 out]
        n91 = property class="VI"(reference=w187) -> ("Panel"=w194:refnum<vi>)  [unwired: 1 in, 2 out]
        n92 = property class="Pnl"(reference=w194) -> (error out=w191:errorcluster, "Controls[]"=w193:refnum<vi>[])  [unwired: 1 in, 1 out]
        n93 = for {
          tunnel: w193 -> [w201] mode=indexing
          tunnel: "Boolean Text" -> [w198]
          tunnel: w191 -> [w196]
          tunnel: [w197] -> w192 mode=indexing
          w199 = refnum<vi> refnum  # Boolean
          n94 = To More Specific Class(target class=w199, reference=w201, error in=w196) -> (specific class reference=w200:refnum<vi>, error out=w195:errorcluster)
          n95 = property class="Bool"(reference=w200, error in=w195, "BoolText.Text"=w198) -> (error out=w197:errorcluster)  [unwired: 1 out]
        }
        n96 = Merge Errors(w192) -> (w189:errorcluster)
        n97 = invoke class="VI" method="Save.Instrument"(reference=w187, error in=w189) -> (error out=w188:errorcluster)  [unwired: 4 in, 5 out]
      }
      event "Button Size", "update button size": Value Change {
        w208 = refnum<vi> refnum  # Boolean
        n98 = event-data() -> ()  [unwired: 1 in, 1 out]
        n99 = property class="VI"(reference=w207) -> ("Panel"=w211:refnum<vi>)  [unwired: 1 in, 2 out]
        n100 = property class="Pnl"(reference=w211) -> ("Controls[]"=w206:refnum<vi>[])  [unwired: 1 in, 2 out]
        n101 = Index Array(array=w206) -> (element=w210:refnum<vi>)  [unwired: 1 in]
        n102 = To More Specific Class(target class=w208, reference=w210) -> (specific class reference=w209:refnum<vi>)  [unwired: 1 in, 1 out]
        n103 = property class="Bool"(reference=w209, "Button Size"="Button Size") -> (error out=w205:errorcluster)  [unwired: 1 in, 1 out]
      }
      event "update button text location", "Button Text Location": Value Change {
        w220 = refnum<vi> refnum  # Boolean
        n104 = event-data() -> ()  [unwired: 1 in, 6 out]
        n105 = property class="VI"(reference=w219) -> ("Panel"=w223:refnum<vi>)  [unwired: 1 in, 2 out]
        n106 = property class="Pnl"(reference=w223) -> ("Controls[]"=w218:refnum<vi>[])  [unwired: 1 in, 2 out]
        n107 = Index Array(array=w218) -> (element=w222:refnum<vi>)  [unwired: 1 in]
        n108 = To More Specific Class(target class=w220, reference=w222) -> (specific class reference=w221:refnum<vi>)  [unwired: 1 in, 1 out]
        n109 = Add(x="Button Text Location", y=cluster{"Left":i32, "Top":i32} {"Left"=0, "Top"=0}) -> (x+y=w215:cluster{"Left":i32, "Top":i32})
        n110 = property class="Bool"(reference=w221, "BoolText.Position"=w215) -> (error out=w217:errorcluster)  [unwired: 1 in, 1 out]
      }
      event "Boolean Text Format", "update text format": Value Change {
        n111 = event-data() -> ()  [unwired: 1 in, 1 out]
        n112 = property class="VI"(reference=w231) -> ("Panel"=w237:refnum<vi>)  [unwired: 1 in, 2 out]
        n113 = Unbundle By Name("Boolean Text Format") -> ("Font:Color"=w229:u32, "Font:Bold?"=w228:bool, "Font:Name"=w227:string, "Font:Size"=w226:u32)
        n114 = property class="Pnl"(reference=w237) -> (error out=w234:errorcluster, "Controls[]"=w236:refnum<vi>[])  [unwired: 1 in, 1 out]
        n115 = for {
          tunnel: w236 -> [w247] mode=indexing
          tunnel: w229 -> [w241]
          tunnel: w234 -> [w243]
          tunnel: [w244] -> w235 mode=indexing
          tunnel: w228 -> [w240]
          tunnel: w227 -> [w239]
          tunnel: w226 -> [w238]
          w245 = refnum<vi> refnum  # Boolean
          n116 = To More Specific Class(target class=w245, reference=w247, error in=w243) -> (specific class reference=w246:refnum<vi>, error out=w242:errorcluster)
          n117 = property class="Bool"(reference=w246, error in=w242, "BoolText.FontColor"=w241, "BoolText.TextColor"=w241, "BoolText.FontBold"=w240, "BoolText.FontName"=w239, "BoolText.FontSize"=w238) -> (error out=w244:errorcluster)  [unwired: 1 out]
        }
        n118 = Merge Errors(w235) -> (w233:errorcluster)
        n119 = invoke class="VI" method="Save.Instrument"(reference=w231, error in=w233) -> (error out=w232:errorcluster)  [unwired: 4 in, 5 out]
      }
      event "Save": Value Change {
        n120 = event-data() -> ()  [unwired: 1 in, 1 out]
        n121 = call "File Dialog"("pattern (all files)"="*.ctl" ("pattern label")) -> ("selected path"=w251:path, "error out"=w252:errorcluster)  [unwired: 11 in, 2 out]
        n122 = property class="VI"(reference=w256) -> ("Panel"=w257:refnum<vi>)  [unwired: 1 in, 2 out]
        n123 = property class="Pnl"(reference=w257) -> ("Controls[]"=w255:refnum<vi>[])  [unwired: 1 in, 2 out]
        n124 = Index Array(array=w255) -> (element=w254:refnum<vi>)  [unwired: 1 in]
        n125 = case shown="No Error" w252 {
          selector: w252 -> [w268 w278]
          tunnel: w254 -> [w273 _]
          tunnel: [w270 w277] -> w253
          tunnel: w251 -> [w267 _]
          frame No Error {
            w262 = TRUE  # Is Persistent?
            # "save as a .ctl file with the tag data applied for the control-level"
            n126 = New VI(8:w268, 9:T5."Control VI" ("vi type (standard vi)")) -> (0:w275:errorcluster, 3:w274:refnum<vi>)  [unwired: 5 in]
            n127 = invoke class="VI" method="Create from Reference"(reference=w274, error in=w275, "Source Object Ref"=w273) -> (reference out=w264:refnum<vi>, error out=w272:errorcluster, "New Object Ref"=w266:refnum<vi>)  [unwired: 4 in, 4 out]
            n128 = property on="Color Level" class="Ring (strict)"() -> ("RingText.Text"=w258:string)  [unwired: 2 in, 2 out]
            n129 = property class="Ctl"(reference=w266, error in=w272, "Position"=T4 {"Left"=24, "Top"=24}) -> (reference out=w260:refnum<vi>, error out=w261:errorcluster)
            n130 = invoke class="Ctl" method="Tag.Set Tag"(reference=w260, error in=w261, "TagName"="control-level" ("Tag Name"), "Value"=w258, "isPersistent"=w262) -> (error out=w259:errorcluster)  [unwired: 2 in, 6 out]
            n131 = invoke class="VI" method="Save.Instrument"(reference=w264, error in=w259, "Path to saved file"=w267) -> (reference out=w269:refnum<vi>, error out=w271:errorcluster)  [unwired: 3 in, 4 out]
            n132 = Close Reference(reference=w269, error in (no error)=w271) -> (error out=w270:errorcluster)
          }
          frame Error {
            n133 = Unbundle By Name(w278) -> ("code"=w279:i32)
            n134 = case shown="Default" w279 {
              tunnel: w278 -> [_ w280]
              tunnel: [_ w280] -> w277
              frame 43 {
              }
              frame Default {
              }
            }
          }
        }
      }
      event Menu Selection (User) {
        n135 = event-data() -> ("ItemTag"=w281:string)  [unwired: 1 in]
        n136 = case shown="\"save\"" w281 {
          tunnel: w285 -> [_ w292]
          tunnel: [_ w289] -> w284
          frame Default {
          }
          frame "save" {
            # "Ctrl+S menu shortcut"
            n137 = call "File Dialog3"("pattern (all files)"="*.ctl" ("pattern label")) -> ("selected path"=w287:path, "error out"=w288:errorcluster)  [unwired: 11 in, 2 out]
            n138 = property class="VI"(reference=w292) -> ("Panel"=w293:refnum<vi>)  [unwired: 1 in, 2 out]
            n139 = property class="Pnl"(reference=w293) -> ("Controls[]"=w291:refnum<vi>[])  [unwired: 1 in, 2 out]
            n140 = Index Array(array=w291) -> (element=w290:refnum<vi>)  [unwired: 1 in]
            n141 = case shown="No Error" w288 {
              selector: w288 -> [w304 w314]
              tunnel: w290 -> [w309 _]
              tunnel: [w306 w313] -> w289
              tunnel: w287 -> [w303 _]
              frame No Error {
                n142 = New VI(8:w304, 9:T5."Control VI" ("vi type (standard vi)")) -> (0:w311:errorcluster, 3:w310:refnum<vi>)  [unwired: 5 in]
                n143 = invoke class="VI" method="Create from Reference"(reference=w310, error in=w311, "Source Object Ref"=w309) -> (reference out=w300:refnum<vi>, error out=w308:errorcluster, "New Object Ref"=w302:refnum<vi>)  [unwired: 4 in, 4 out]
                n144 = property on="Color Level" class="Ring (strict)"() -> ("RingText.Text"=w299:string)  [unwired: 2 in, 2 out]
                n145 = property class="Ctl"(reference=w302, error in=w308, "Position"=T4 {"Left"=24, "Top"=24}) -> (reference out=w295:refnum<vi>, error out=w296:errorcluster)
                n146 = invoke class="Ctl" method="Tag.Set Tag"(reference=w295, error in=w296, "TagName"="control-level" ("Tag Name"), "Value"=w299, "isPersistent"=TRUE ("Is Persistent?")) -> (error out=w294:errorcluster)  [unwired: 2 in, 6 out]
                n147 = invoke class="VI" method="Save.Instrument"(reference=w300, error in=w294, "Path to saved file"=w303) -> (reference out=w305:refnum<vi>, error out=w307:errorcluster)  [unwired: 3 in, 4 out]
                n148 = Close Reference(reference=w305, error in (no error)=w307) -> (error out=w306:errorcluster)
              }
              frame Error {
                n149 = Unbundle By Name(w314) -> ("code"=w315:i32)
                n150 = case shown="43" w315 {
                  tunnel: w314 -> [_ w316]
                  tunnel: [_ w316] -> w313
                  frame 43 {
                  }
                  frame Default {
                  }
                }
              }
            }
          }
        }
      }
      event "Button Type": Value Change {
        w334 = FALSE ("Wait Until Done")
        # "rerun and reinsert VI with new control"
        # "open the selected ctl and replace old one"
        # "abort and remove temporarily"
        # "copy at the start\nso that the original stays unmodified"
        n151 = event-data() -> ()  [unwired: 1 in, 1 out]
        n152 = invoke class="VI" method="Abort VI"(reference=w339) -> (error out=w325:errorcluster)  [unwired: 2 in, 2 out]
        n153 = Strip Path(path=w331) -> (stripped path=w346:path)  [unwired: 1 out]
        n154 = List Folder(path=w346, pattern="*.ctl") -> (path out=w343:path, filenames=w344:string[])  [unwired: 2 in, 2 out]
        n155 = invoke on="Sub Panel" class="SubPnl" method="Remove VI"(error in=w325) -> (error out=w324:errorcluster)  [unwired: 2 in, 2 out]
        n156 = Index Array(array=w344, index="Button Type") -> (element=w342:string)
        n157 = Unbundle By Name(w319) -> ("update colors"=w318:refnum<user-event>)
        n158 = Build Path(base path=w343, name or relative path=w342) -> (appended path=w340:path)
        n159 = call <vilib>:"Clear Errors.vi"("error in (no error)"=w324) -> ("error out"=w323:errorcluster)  [unwired: 5 in, 1 out]
        n160 = property class="VI"(reference=w339, error in=w323) -> (reference out=w321:refnum<vi>, error out=w328:errorcluster, "Panel"=w348:refnum<vi>)
        n161 = Generate User Event(user event=w318, event data cluster=variant ("event data")) -> ()  [unwired: 2 in, 2 out]
        n162 = property class="Pnl"(reference=w348, error in=w328) -> (error out=w327:errorcluster, "Controls[]"=w347:refnum<vi>[])  [unwired: 1 out]
        n163 = Index Array(array=w347) -> (element=w341:refnum<vi>)  [unwired: 1 in]
        n164 = invoke class="Ctl" method="Replace No Attrib"(reference=w341, error in=w327, "Param 1"=w340) -> (error out=w329:errorcluster)  [unwired: 3 in, 5 out]
        n165 = invoke class="VI" method="Save.Instrument"(reference=w321, error in=w329) -> (error out=w322:errorcluster)  [unwired: 4 in, 5 out]
        n166 = Close Reference(reference=w321, error in (no error)=w322) -> (error out=w330:errorcluster)
        n167 = Open VI Reference(vi path=w331, error in (no error)=w330) -> (vi reference=w335:refnum<vi>, error out=w336:errorcluster)  [unwired: 4 in]
        n168 = local read "Decal Image"() -> (w320:path)
        n169 = invoke class="VI" method="Run VI"(reference=w335, error in=w336, "Wait until done"=w334, "Auto Dispose Ref"=w334) -> (reference out=w332:refnum<vi>, error out=w326:errorcluster)  [unwired: 1 in, 3 out]
        n170 = property on="Decal Image" class="Path"("Val(Sgnl)"=w320) -> ()  [unwired: 2 in, 2 out]
        n171 = invoke on="Sub Panel" class="SubPnl" method="Insert VI"(error in=w326, "VI Ref"=w332) -> (error out=w333:errorcluster)  [unwired: 2 in, 3 out]
      }
      event "Open": Value Change {
        n172 = event-data() -> ()  [unwired: 1 in, 1 out]
        n173 = call "File Dialog2"("pattern label"="*.ctl") -> ("selected path"=w351:path, "error out"=w353:errorcluster)  [unwired: 11 in, 2 out]
        n174 = case shown="No Error" w353 {
          selector: w353 -> [w371 w405]
          tunnel: [w357 w404] -> w352
          tunnel: w351 -> [w362 _]
          tunnel: w350 -> [w370 _]
          frame No Error {
            w397 = refnum<vi> refnum  # Boolean
            # "#update later"
            n175 = invoke class="VI" method="Abort VI"(reference=w370, error in=w371) -> (reference out=w360:refnum<vi>, error out=w372:errorcluster)  [unwired: 1 in, 1 out]
            n176 = Close Reference(reference=w360, error in (no error)=w372) -> (error out=w361:errorcluster)
            n177 = call <vilib>:"Clear Errors.vi"("error in (no error)"=w361) -> ("error out"=w358:errorcluster)  [unwired: 5 in, 1 out]
            n178 = Open VI Reference(vi path=w362, error in (no error)=w358) -> (vi reference=w396:refnum<vi>, error out=w395:errorcluster)  [unwired: 4 in]
            n179 = property class="VI"(reference=w396, error in=w395) -> (reference out=w392:refnum<vi>, error out=w394:errorcluster, "Panel"=w398:refnum<vi>)
            n180 = property class="Pnl"(reference=w398, error in=w394) -> (error out=w393:errorcluster, "Controls[]"=w401:refnum<vi>[])  [unwired: 1 out]
            n181 = Index Array(array=w401) -> (element=w399:refnum<vi>)  [unwired: 1 in]
            n182 = To More Specific Class(target class=w397, reference=w399, error in=w393) -> (specific class reference=w400:refnum<vi>, error out=w368:errorcluster)
            n183 = property class="Bool"(reference=w400, error in=w368) -> (error out=w391:errorcluster, "Position"=w364:T4, "Label.Height"=w365:u32, "Button Size"=w389:T6, "BoolText.Text"=w388:string, "BoolText.TextColor"=w387:u32, "BoolText.FontBold"=w386:bool, "BoolText.FontName"=w385:string, "BoolText.FontSize"=w384:u32, "Colors [4]"=w379:cluster{u32, u32}[])  [unwired: 1 out]
            n184 = Index Array(array=w379) -> (element #1=w378:cluster{u32, u32}, element #2=w377:cluster{u32, u32}, element #3=w376:cluster{u32, u32}, element #4=w375:cluster{u32, u32}, element #5=w374:cluster{u32, u32}, element #6=w373:cluster{u32, u32})  [unwired: 6 in]
            n185 = Close Reference(reference=w392, error in (no error)=w391) -> (error out=w359:errorcluster)
            n186 = call "Update Custom UI for Button.vi"("error in"=w359, "selected path"=w362) -> ("error out"=w369:errorcluster, "appended path"=w363:path)  [unwired: 8 in]
            n187 = Bundle By Name(cluster=T2 {"false color"={"border"=15922170, "fill"=15922170}, "true color"={"border"=14936305, "fill"=14936305}, "click false color"={"border"=14410221, "fill"=14410221}, "click true color"={"border"=14410221, "fill"=14410221}, "hover false color"={"border"=14540516, "fill"=14540516}, "hover true color"={"border"=14540516, "fill"=14540516}} ("Boolean Colors"), "false color"=w378, "true color"=w377, "click true color"=w376, "click false color"=w375, "hover false color"=w374, "hover true color"=w373) -> (w380:T2)
            n188 = Unbundle By Name(w364) -> ("Top"=w367:i32)
            n189 = Bundle By Name(cluster=T1 {"Font:Color"=3563918, "Font:Bold?"=TRUE, "Font:Name"="App Font", "Font:Size"=22} ("Boolean Text Format"), "Font:Color"=w387, "Font:Bold?"=w386, "Font:Name"=w385, "Font:Size"=w384) -> (w383:T1)
            n190 = Add(x=w367, y=w365) -> (x+y=w366:u32)
            n191 = Bundle By Name(cluster=w364, "Top"=w366) -> ()  [unwired: 1 out]
            n192 = flat-sequence {
              tunnel: w363 -> [w403]
              tunnel: [w402] -> w356
              tunnel: w369 -> [_]
              frame #0 {
                n193 = call "Read Image on Button.vi"("File with Button"=w403) -> ("png file out"=w402:path)  [unwired: 9 in, 1 out]
              }
            }
            n194 = property on="Button Type" class="Ring (strict)"(error in=w369, "Val(Sgnl)"=u16 5 ("Value (Signaling)")) -> (error out=w357:errorcluster)  [unwired: 1 in, 1 out]
            n195 = local write "Button Size"(w389) -> ()
            n196 = local write "Boolean Text"(w388) -> ()
            n197 = local write "Boolean Colors"(w380) -> ()
            n198 = local write "Boolean Text Format"(w383) -> ()
            n199 = local write "Decal Image"(w356) -> ()
          }
          frame Error {
            n200 = Unbundle By Name(w405) -> ("code"=w406:i32)
            n201 = case shown="Default" w406 {
              tunnel: w405 -> [w407 _]
              tunnel: [w407 _] -> w404
              frame Default {
              }
              frame 43 {
              }
            }
          }
        }
      }
    }
    "error out" <- w24
    n202 = call <vilib>:"Simple Error Handler.vi"("error in (no error)"=w24) -> ()  [unwired: 4 in, 5 out]
  }
  n203 = call "User Event Close.vi"("Event Registration Refnum"=w14, "user events"=w13) -> ()  [unwired: 9 in, 1 out]
  n204 = flat-sequence {
    tunnel: w20 -> [_]
    frame #0 {
      n205 = disable-structure shown="Disabled" {
        frame Disabled {
          n206 = control-ref of="This VI"() -> (w408:refnum<vi>)
          n207 = invoke class="VI" method="FP.Close"(reference=w408) -> ()  [unwired: 2 in, 3 out]
        }
        frame Enabled {
        }
      }
    }
  }
  n208 = invoke class="VI" method="Abort VI"(reference=w20) -> (reference out=w23:refnum<vi>, error out=w22:errorcluster)  [unwired: 2 in, 1 out]
  n209 = Close Reference(reference=w23, error in (no error)=w22) -> ()  [unwired: 1 out]
